vi "Oszi_Offset_Messen.vi"(8 "Error_in":errorcluster, 10 "Channel":i32=1, 11 "VISA Name OZ in(OZ)":refnum<visa-resource-name>="USB0::0x0957::0x179B::MY54313507::INSTR") -> (0 "Error_out":errorcluster, 2 "Offset_Spannung":dbl, 3 "VISA Name OZ out":refnum<visa-resource-name>="USB0::0x0957::0x179B::MY54313507::INSTR")   [LabVIEW 2016]
doc: "Mit diesem VI kann der Offset des Oszilloscopes aus den Messdaten herrausgerechnet werden."
panel:
  out "Ausgangs-String":string
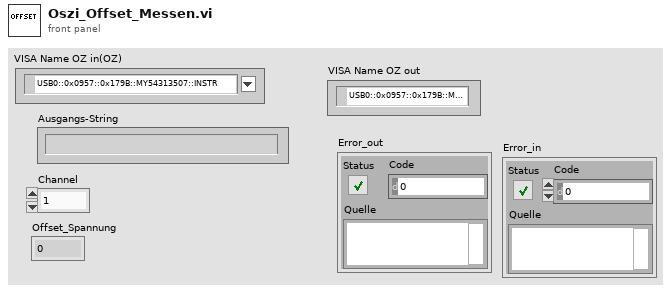
[diagram p1: front panel]
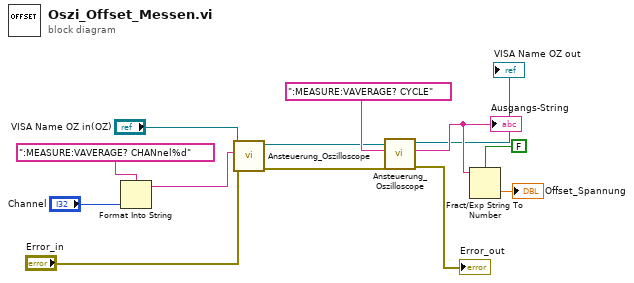
[diagram p0: block diagram]
diagram:
  n1 = Format Into String(format string=":MEASURE:VAVERAGE? CHANnel%d" ("Eingangs-String"), "Channel") -> (resulting string=w1:string)  [unwired: 2 in, 1 out]
  n2 = call "Ansteuerung_Oszilloscope.vi"("Error_in"="Error_in", "Eingangs-String"=w1, "VISA Name OZ in(OZ)"="VISA Name OZ in(OZ)") -> ("Error_out"=w12:errorcluster, "VISA Name OZ out"=w10:refnum<visa-resource-name>)  [unwired: 6 in, 1 out]
  n3 = call "Ansteuerung_Oszilloscope.vi"("Error_in"=w12, "Eingangs-String"=":MEASURE:VAVERAGE? CYCLE", "VISA Name OZ in(OZ)"=w10) -> ("Error_out"=→"Error_out":errorcluster, "Ausgangs-String"=w9:string, "VISA Name OZ out"=→"VISA Name OZ out":refnum<visa-resource-name>)  [unwired: 6 in]
  "Ausgangs-String" <- w9
  n4 = Fract/Exp String To Number(use system decimal point (T)=FALSE ("Systemdezimalzeichen verwenden (T)"), string=w9) -> (number=→"Offset_Spannung":dbl)  [unwired: 2 in, 1 out]
